vi "New Terminals Updated_1.vi"(7 "Prev Terminal Count":u32, 8 "error in (no error)":errorcluster, 9 "Analytics Button Pressed?":bool, 10 "Samples to display":i32, 11 "Terminal Count":u32) -> (0 "error out":errorcluster, 1 "Top/Bottom":bool, 2 "Values Inserted":u32, 3 "No Of New Terminals":u32, 5 "Prev Terminal Count":u32)   [LabVIEW 2019, in "Zen Analytics.lvlib" / "Zen Analytics.lvclass"]
uses:
  Zen Analytics.lvclass
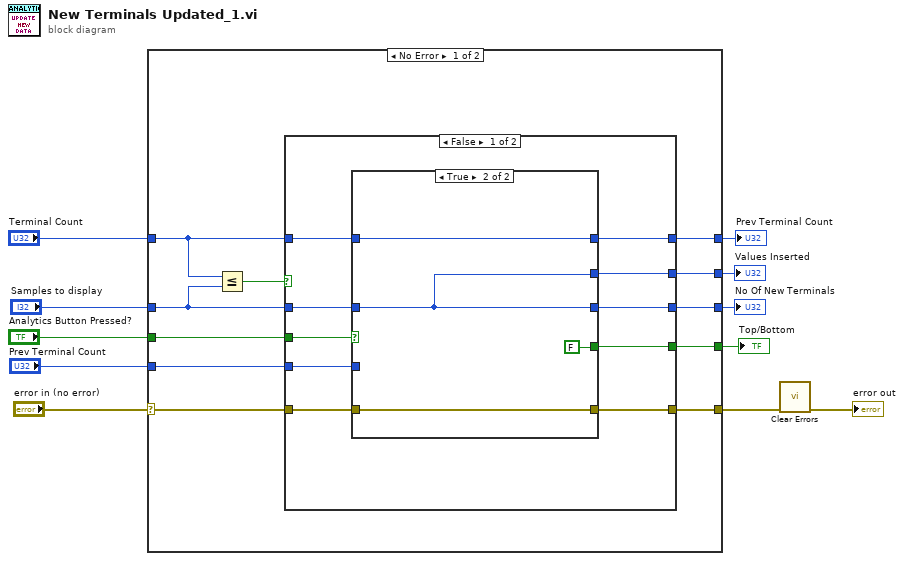
[diagram p0: block diagram]
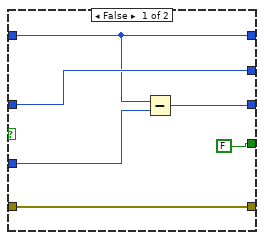
[diagram p2: hidden frame]
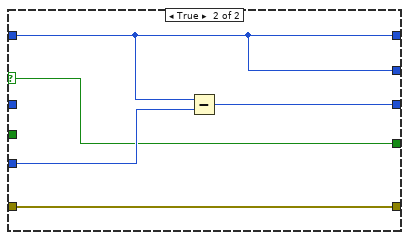
[diagram p3: hidden frame]
diagram:
  n1 = case shown="No Error" "error in (no error)" {
    selector: "error in (no error)" -> [w22 w52]
    tunnel: [w21 w52] -> w2
    tunnel: "Analytics Button Pressed?" -> [w20 w50]
    tunnel: [w19 w51] -> w9
    tunnel: "Prev Terminal Count" -> [w18 w51]
    tunnel: [w17 w49] -> w7
    tunnel: "Terminal Count" -> [w14 w49]
    tunnel: "Samples to display" -> [w13 w48]
    tunnel: [w16 w50] -> w4
    tunnel: [w12 w48] -> w3
    frame No Error {
      n2 = Less Or Equal?(x=w14, y=w13) -> (x <= y?=w15:bool)
      n3 = case shown="False" w15 {
        selector: w15 -> [_ w43]
        tunnel: w22 -> [w32 w47]
        tunnel: [w31 w47] -> w21
        tunnel: w20 -> [w30 _]
        tunnel: [w29 w45] -> w19
        tunnel: w18 -> [w28 w46]
        tunnel: [w27 w44] -> w17
        tunnel: w14 -> [w23 w44]
        tunnel: w13 -> [w26 _]
        tunnel: [w25 w43] -> w16
        tunnel: [w24 w44] -> w12
        frame False {
          n4 = case shown="True" w30 {
            tunnel: w32 -> [w36 w42]
            tunnel: [w36 w42] -> w31
            tunnel: [w37 w41] -> w29
            tunnel: [w34 w40] -> w27
            tunnel: w28 -> [w38 _]
            tunnel: w26 -> [w35 w41]
            tunnel: [FALSE FALSE] -> w25
            tunnel: [w35 w41] -> w24
            tunnel: w23 -> [w34 w40]
            frame False {
              n5 = Subtract(x=w34, y=w38) -> (x-y=w37:u32)
            }
            frame True {
            }
          }
        }
        frame True {
          n6 = Subtract(x=w44, y=w46) -> (x-y=w45:u32)
        }
      }
    }
    frame Error {
    }
  }
  "No Of New Terminals" <- w9
  "Prev Terminal Count" <- w7
  "Top/Bottom" <- w4
  "Values Inserted" <- w3
  n7 = call <vilib>:"Clear Errors.vi"("error in (no error)"=w2) -> ("error out"=→"error out":errorcluster)  [unwired: 5 in, 1 out]
